vi "test Update State Value.vi"(8 "error in (no error)":errorcluster, 11 "TestCase in":refnum<class "Routing and Faulting State Value Table Unit Tests.lvclass">) -> (0 "error out":errorcluster, 3 "TestCase out":refnum<class "Routing and Faulting State Value Table Unit Tests.lvclass">)   [LabVIEW 2019, in "Routing and Faulting State Value Table Unit Tests.lvclass"]
uses:
  Routing and Faulting State Value Table Unit Tests.lvclass
  System Explorer/State-Value Row.ctl
  Shared/Channel States.ctl
  Shared/Routing State.ctl
  Shared/Connection.ctl
  Routing and Faulting State Value Table Unit Tests.lvclass/Routing and Faulting State Value Table Unit Tests.ctl
  <vilib>/addons/_JKI Toolkits/VI Tester/TestCase.llb/TestCase.lvclass
  System Explorer/Routing and Faulting System Explorer.lvlib
  Shared/Routing and Faulting Shared.lvlib
  Scripting/Routing and Faulting Scripting.lvlib
  C:/Program Files (x86)/National Instruments/LabVIEW 2019/vi.lib/addons/_JKI Toolkits/VI Tester/TestCase.llb/TestCase.lvclass
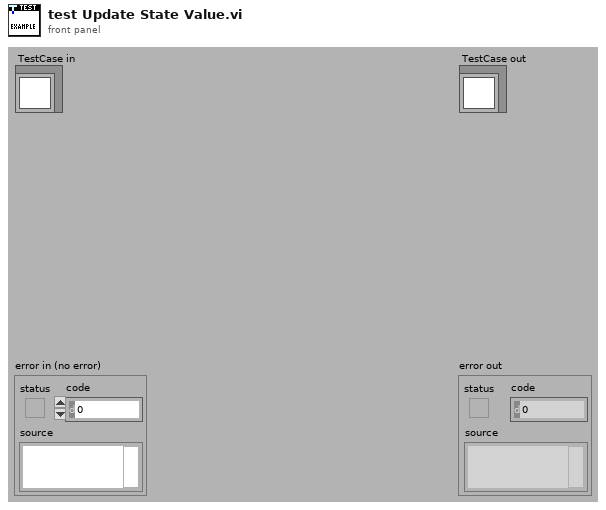
[diagram p1: front panel]
types:
  T1 = typedef "Routing and Faulting Shared.lvlib/Channel States.ctl" = T2[]
  T2 = typedef "Routing and Faulting Shared.lvlib/Routing State.ctl" = cluster{"Name":string, "Description":string, "Value":i32, "Connection List":T3[]}
  T3 = typedef "Routing and Faulting Shared.lvlib/Connection.ctl" = cluster{"Module":string, "Source":string, "Destination":string}
  T4 = typedef "Routing and Faulting System Explorer.lvlib/State-Value Row.ctl" = cluster{"State":string, "State Value":string}
  T5 = typedef "Custom Device API.lvlib/Custom Device Item Ref.ctl" = u64
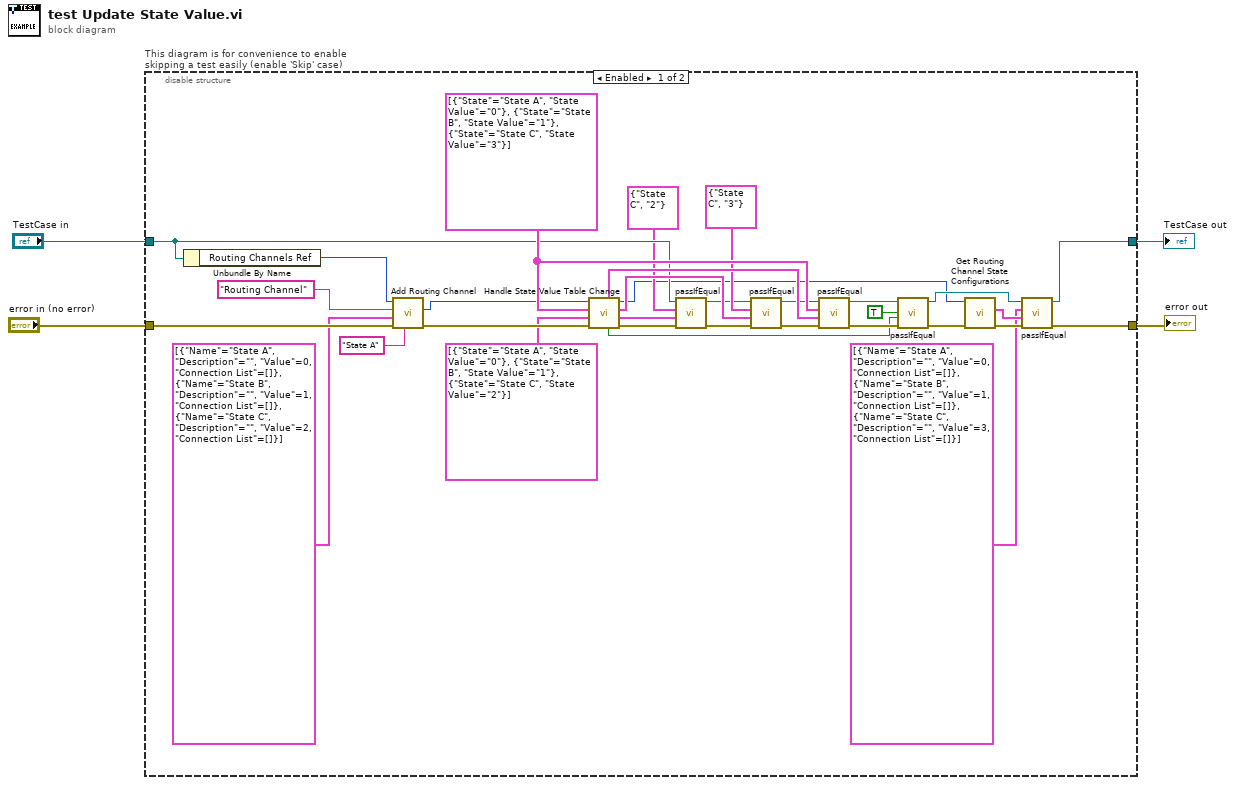
[diagram p0: block diagram]
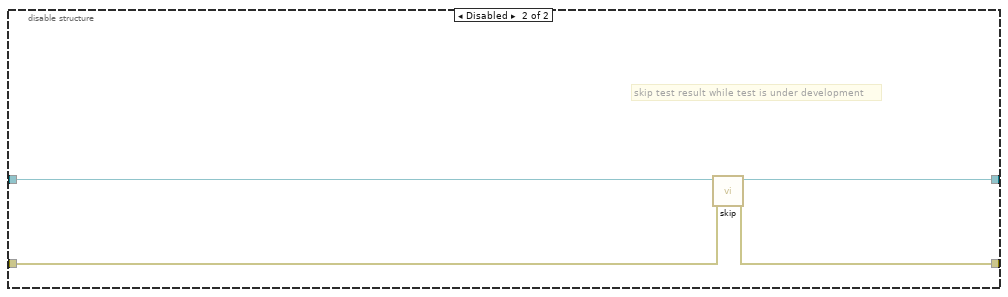
[diagram p2: hidden frame]
diagram:
  n1 = disable-structure "This diagram is for convenience to enable skipping a test easily (enable 'Skip' case)" shown="Enabled" {
    disable-tunnel: "TestCase in" -> [w19 w40]
    disable-tunnel: [w9 w38] -> w1
    disable-tunnel: [w10 w39] -> w3
    disable-tunnel: "error in (no error)" -> [w36 w37]
    frame Enabled {
      w29 = T4[] [{"State"="State A", "State Value"="0"}, {"State"="State B", "State Value"="1"}, {"State"="State C", "State Value"="3"}] ("NewVal")
      n2 = Unbundle By Name(w19) -> ("Routing Channels Ref"=w34:T5)
      n3 = call "Add Routing Channel.vi"("initial state"="State A", "error in"=w36, "state configurations"=T1 [{"Name"="State A", "Description"="", "Value"=0, "Connection List"=[]}, {"Name"="State B", "Description"="", "Value"=1, "Connection List"=[]}, {"Name"="State C", "Description"="", "Value"=2, "Connection List"=[]}], "channel name"="Routing Channel", "routing channels in"=w34) -> ("error out"=w35:errorcluster, "routing channel"=w26:T5)  [unwired: 4 in, 1 out]
      n4 = call "Handle State Value Table Change.vi"("error in (no error)"=w35, "OldVal"=T4[] [{"State"="State A", "State Value"="0"}, {"State"="State B", "State Value"="1"}, {"State"="State C", "State Value"="2"}] ("NewVal"), "NewVal"=w29, "routing channel in"=w26) -> ("error out"=w16:errorcluster, "old modified state and value"=w20:T4, "new modified state and value"=w23:T4, "routing channel out"=w6:T5, "update controls"=w14:bool, "coerced newval"=w30:T4[])  [unwired: 2 in]
      n5 = call-dynamic "passIfEqual.vi"("error in (no error)"=w16, "y"=w20, "x"=T4 {"State"="State C", "State Value"="2"} ("old modified state and value"), "TestCase in"=w19) -> ("error out"=w21:errorcluster, "TestCase out"=w18:refnum<class "Routing and Faulting State Value Table Unit Tests.lvclass">)  [unwired: 6 in]
      n6 = call-dynamic "passIfEqual.vi"("error in (no error)"=w21, "y"=w23, "x"=T4 {"State"="State C", "State Value"="3"} ("new modified state and value"), "TestCase in"=w18) -> ("error out"=w25:errorcluster, "TestCase out"=w24:refnum<class "Routing and Faulting State Value Table Unit Tests.lvclass">)  [unwired: 6 in]
      n7 = call-dynamic "passIfEqual.vi"("error in (no error)"=w25, "y"=w30, "x"=w29, "TestCase in"=w24) -> ("error out"=w32:errorcluster, "TestCase out"=w15:refnum<class "Routing and Faulting State Value Table Unit Tests.lvclass">)  [unwired: 6 in]
      n8 = call-dynamic "passIfEqual.vi"("error in (no error)"=w32, "y"=w14, "x"=TRUE ("update controls"), "TestCase in"=w15) -> ("error out"=w7:errorcluster, "TestCase out"=w8:refnum<class "Routing and Faulting State Value Table Unit Tests.lvclass">)  [unwired: 6 in]
      n9 = call "Get Routing Channel State Configurations.vi"("error in"=w7, "routing channel in"=w6) -> ("error out"=w12:errorcluster, "state configurations"=w11:T1)  [unwired: 7 in, 1 out]
      n10 = call-dynamic "passIfEqual.vi"("error in (no error)"=w12, "y"=w11, "x"=T1 [{"Name"="State A", "Description"="", "Value"=0, "Connection List"=[]}, {"Name"="State B", "Description"="", "Value"=1, "Connection List"=[]}, {"Name"="State C", "Description"="", "Value"=3, "Connection List"=[]}] ("state configurations"), "TestCase in"=w8) -> ("error out"=w10:errorcluster, "TestCase out"=w9:refnum<class "Routing and Faulting State Value Table Unit Tests.lvclass">)  [unwired: 6 in]
    }
    frame Disabled {
      # "skip test result while test is under development"
      n11 = call <vilib>:"skip.vi"("error in (no error)"=w37, "TestCase in"=w40) -> ("error out"=w39:errorcluster, "TestCase out"=w38:refnum<class "Routing and Faulting State Value Table Unit Tests.lvclass">)  [unwired: 8 in]
    }
  }
  "error out" <- w3
  "TestCase out" <- w1
